vi "Amiee's latency characterization try1.vi"() -> ()   [LabVIEW 2016]
uses:
  <vilib>/DAQmx/write.llb/DAQmx Write (Digital Bool 1Line 1Point).vi
  <vilib>/DAQmx/read.llb/DAQmx Read (Digital Bool 1Line 1Point).vi
  <vilib>/Utility/file.llb/Write Delimited Spreadsheet (string).vi
  <vilib>/DAQmx/miscellaneous.llb/DAQmx Fill In Error Info.vi
  <vilib>/Utility/file.llb/Write Delimited Spreadsheet (I64).vi
panel:
  out "Delay (ms)":u32
  out "tock":u32
  out "tick":u32
  in  "stop":bool
  out "Waiting?":bool
  in  "output \nto robit":bool
  # "Latency Characterization\nAuthor: Amiee Jackson, Aaron Thornton, Brian Post (08/2017)\nObjective: Let LabView flag an output to the robot through the PXI, \nwhere the robot, upon receiving this flag, will immediately respond \nwith a flag back to LabView.  Write this data to a tab-delimited text file."
  # "Instructions:\nPress \"run\" to begin a cycle.\nPress \"stop\" to stop."
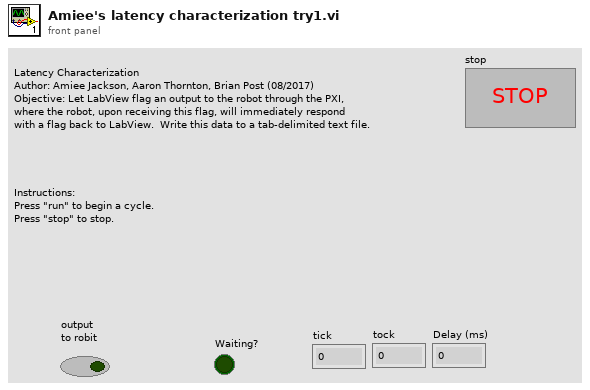
[diagram p1: front panel]
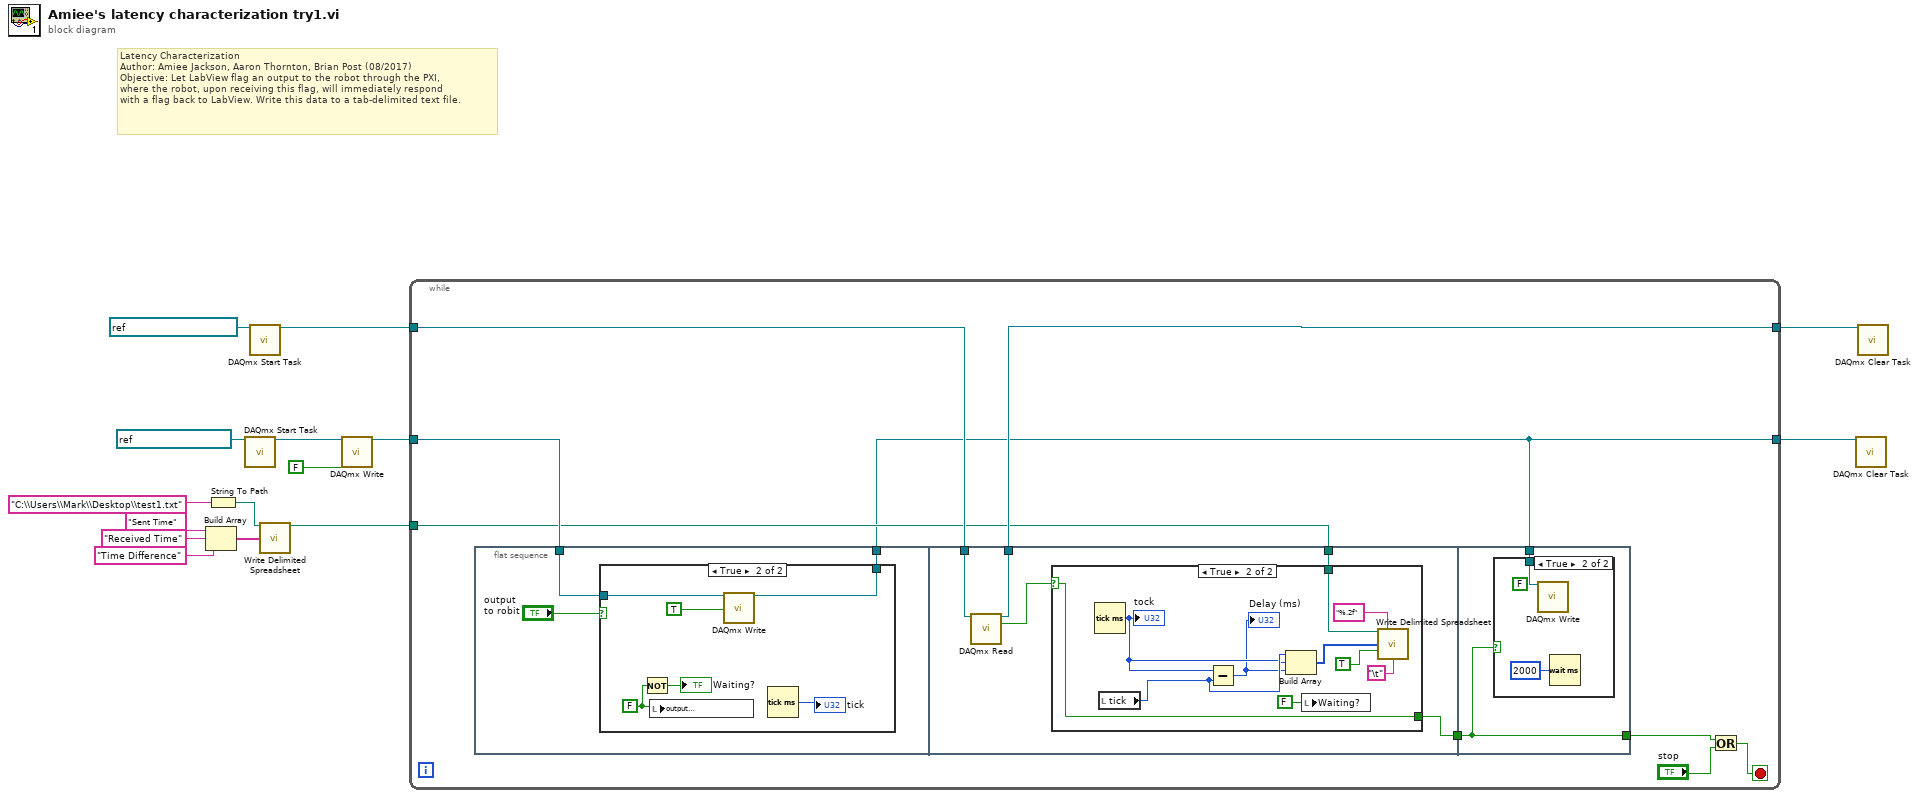
[diagram p0: block diagram]
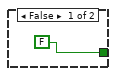
[diagram p3: hidden frame]
diagram:
  # "Latency Characterization\nAuthor: Amiee Jackson, Aaron Thornton, Brian Post (08/2017)\nObjective: Let LabView flag an output to the robot through the PXI, \nwhere the robot, upon receiving this flag, will immediately respond \nwith a flag back to LabView. Write this data to a tab-delimited text file."
  n1 = Build Array("Sent Time", "Received Time", "Time Difference") -> (w12:string[])
  n2 = String To Path(string="C:\\Users\\Mark\\Desktop\\test1.txt") -> (path=w9:path)
  n3 = call <vilib>:"DAQmx Start Task.vi"("task/channels in"=refnum<k21> "KUKA IN 3") -> ("task out"=w2:refnum<k21>)  [unwired: 13 in, 1 out]
  n4 = call <vilib>:"DAQmx Start Task.vi"("task/channels in"=refnum<k21> "KUKA OUT 13") -> ("task out"=w6:refnum<k21>)  [unwired: 13 in, 1 out]
  n5 = call-poly <vilib>:"Write Delimited Spreadsheet.vi"("file path (dialog if empty)"=w9, "1D data"=w12) -> ("new file path (Not A Path if cancelled)"=w11:path)  [unwired: 12 in, 1 out]
  n6 = call-poly <vilib>:"DAQmx Write.vi"("task/channels in"=w2, "data"=FALSE) -> ("task out"=w1:refnum<k21>)  [unwired: 11 in, 2 out]
  n7 = while {
    tunnel: w11 -> [w21]
    tunnel: w1 -> [w24]
    tunnel: w6 -> [w23]
    tunnel: [w22] -> w5
    tunnel: [w16] -> w4
    stop <- w17 stop-if-true
    n8 = flat-sequence {
      tunnel: w24 -> [w26]
      tunnel: [w25] -> w16
      tunnel: w23 -> [w39]
      tunnel: [w38] -> w22
      tunnel: w21 -> [w36]
      tunnel: [w35] -> w20
      tunnel: [w52] -> w19
      tunnel: w20 -> [w52]
      tunnel: w16 -> [w51]
      frame #0 {
        n9 = case shown="True" "output \nto robit" {
          tunnel: w26 -> [w28 w31]
          tunnel: [w28 w30] -> w25
          frame False {
          }
          frame True {
            w33 = FALSE
            n10 = Not(x=w33) -> (.not. x?=→"Waiting?":bool)
            n11 = local write "output \nto robit"(w33) -> ()
            n12 = call-poly <vilib>:"DAQmx Write.vi"("task/channels in"=w31, "data"=TRUE) -> ("task out"=w30:refnum<k21>)  [unwired: 11 in, 2 out]
            n13 = Tick Count (ms)() -> (millisecond timer value=→"tick":u32)
          }
        }
      }
      frame #1 {
        n14 = call-poly <vilib>:"DAQmx Read.vi"("task/channels in"=w39) -> ("task out"=w38:refnum<k21>, "data"=w37:bool)  [unwired: 12 in, 1 out]
        n15 = case shown="True" w37 {
          selector: w37 -> [_ w46]
          tunnel: w36 -> [_ w47]
          tunnel: [FALSE w46] -> w35
          frame False {
          }
          frame True {
            n16 = Tick Count (ms)() -> (millisecond timer value=w44:u32)
            "tock" <- w44
            n17 = local read "tick"() -> (w45:u32)
            n18 = Subtract(x=w44, y=w45) -> (x-y=w43:u32)
            "Delay (ms)" <- w43
            n19 = Build Array(w45, w44, w43) -> (w42:u32[])
            n20 = local write "Waiting?"(FALSE ("Waiting?")) -> ()
            n21 = call-poly <vilib>:"Write Delimited Spreadsheet.vi"("file path (dialog if empty)"=w47, "format (%d)"="%.2f" ("format (%.3f)"), "1D data"=w42, "append to file? (new file:F)"=TRUE, "delimiter (\\t)"="\t") -> ()  [unwired: 9 in, 2 out]
          }
        }
      }
      frame #2 {
        n22 = case shown="True" w52 {
          tunnel: w51 -> [_ w54]
          frame False {
          }
          frame True {
            n23 = call-poly <vilib>:"DAQmx Write.vi"("task/channels in"=w54, "data"=FALSE) -> ()  [unwired: 11 in, 3 out]
            n24 = Wait (ms)(milliseconds to wait=u32 2000) -> ()  [unwired: 1 out]
          }
        }
      }
    }
    n25 = Or(x=w19, y="stop") -> (x .or. y?=w17:bool)
  }
  n26 = call <vilib>:"DAQmx Clear Task.vi"("task in"=w4) -> ()  [unwired: 14 in, 1 out]
  n27 = call <vilib>:"DAQmx Clear Task.vi"("task in"=w5) -> ()  [unwired: 14 in, 1 out]
